vi "[PC]LogSnapshot.vi"(11 "LogFileRef":refnum<k34>) -> ()   [LabVIEW 2018]
uses:
  RT/[GlobVar]SensorState.vi
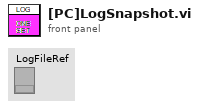
[diagram p1: front panel]
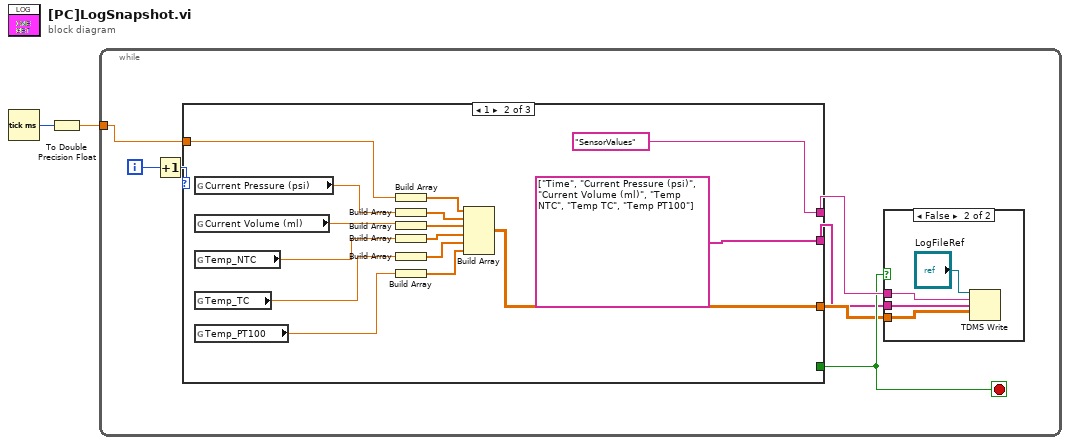
[diagram p0: block diagram]
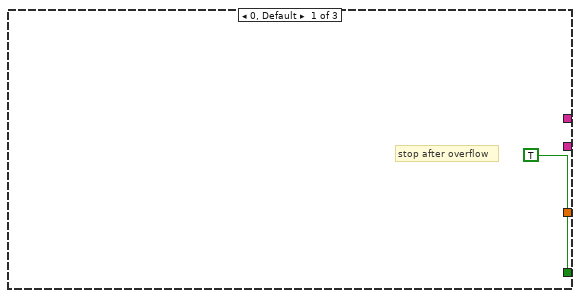
[diagram p3: hidden frame]
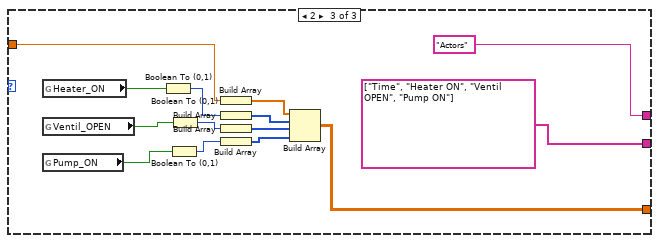
[diagram p4: hidden frame]
diagram:
  n1 = Tick Count (ms)() -> (millisecond timer value=w2:u32)
  n2 = To Double Precision Float(number=w2) -> (double precision float=w1:dbl)
  n3 = while {
    tunnel: w1 -> [w4]
    i -> [w9]
    stop <- w6 stop-if-true
    n4 = Increment(x=w9) -> (x+1=w8:i32)
    n5 = case shown="1" w8 {
      tunnel: [TRUE _ _] -> w6
      tunnel: [_ "SensorValues" ("Gruppenname (Eingang, Unbenannt)") "Actors" ("Gruppenname (Eingang, Unbenannt)")] -> w7
      tunnel: [_ w26 w40] -> w5
      tunnel: w4 -> [_ w25 w39]
      tunnel: [_ string[] ["Time", "Current Pressure (psi)", "Current Volume (ml)", "Temp NTC", "Temp TC", "Temp PT100"] ("Kanalnamen (Eingang, unbenannt)") string[] ["Time", "Heater ON", "Ventil OPEN", "Pump ON"] ("Kanalnamen (Eingang, unbenannt)")] -> w3
      frame 0, Default {
        # "stop after overflow"
      }
      frame 1 {
        n6 = global read "[GlobVar]SensorState.vi" "Current Pressure (psi)"() -> (w24:dbl)
        n7 = global read "[GlobVar]SensorState.vi" "Current Volume (ml)"() -> (w22:dbl)
        n8 = global read "[GlobVar]SensorState.vi" "Temp_NTC"() -> (w20:dbl)
        n9 = global read "[GlobVar]SensorState.vi" "Temp_TC"() -> (w18:dbl)
        n10 = global read "[GlobVar]SensorState.vi" "Temp_PT100"() -> (w17:dbl)
        n11 = Build Array(w25) -> (w28:dbl[])
        n12 = Build Array(w24) -> (w29:dbl[])
        n13 = Build Array(w22) -> (w21:dbl[])
        n14 = Build Array(w20) -> (w19:dbl[])
        n15 = Build Array(w18) -> (w16:dbl[])
        n16 = Build Array(w17) -> (w15:dbl[])
        n17 = Build Array(w28, w29, w21, w19, w16, w15) -> (w26:dbl[][])
      }
      frame 2 {
        n18 = global read "[GlobVar]SensorState.vi" "Heater_ON"() -> (w31:bool)
        n19 = global read "[GlobVar]SensorState.vi" "Ventil_OPEN"() -> (w32:bool)
        n20 = global read "[GlobVar]SensorState.vi" "Pump_ON"() -> (w35:bool)
        n21 = Boolean To (0,1)(Boolean=w31) -> (0, 1=w30:i16)
        n22 = Boolean To (0,1)(Boolean=w35) -> (0, 1=w34:i16)
        n23 = Boolean To (0,1)(Boolean=w32) -> (0, 1=w33:i16)
        n24 = Build Array(w39) -> (w42:dbl[])
        n25 = Build Array(w30) -> (w43:i16[])
        n26 = Build Array(w33) -> (w37:i16[])
        n27 = Build Array(w34) -> (w36:i16[])
        n28 = Build Array(w42, w43, w37, w36) -> (w40:dbl[][])
      }
    }
    n29 = case shown="False" w6 {
      tunnel: w7 -> [_ w13]
      tunnel: w5 -> [_ w12]
      tunnel: w3 -> [_ w11]
      frame True {
      }
      frame False {
        n30 = TDMS Write(0:"LogFileRef", 5:w13, 7:w11, 9:w12) -> ()  [unwired: 2 in, 4 out]
      }
    }
  }
